vi "Oscilloscope Type Axis Scales.vi"(8 "Error In":errorcluster, 9 "Oscilloscope vertical":T1=[{"Volts/Div "=0.5, "Coupling"=enum."DC 1MOhm", "Offset [V]"=0.0, "Channel"=enum."Channel 1"}, {"Volts/Div "=0.2, "Coupling"=enum."DC 1MOhm", "Offset [V]"=0.0, "Channel"=enum."Channel 2"}] {"Offset [V]" format="%#_13p"; "Volts/Div" min=0.001 max=5.0 format="%#_6p"}, 11 "Graph In":refnum<vi>) -> (0 "Error Out":errorcluster, 3 "Graph Out":refnum<vi>)   [LabVIEW 2017]
uses:
  LC93xx HSN/LeC93xx Vertical.ctl
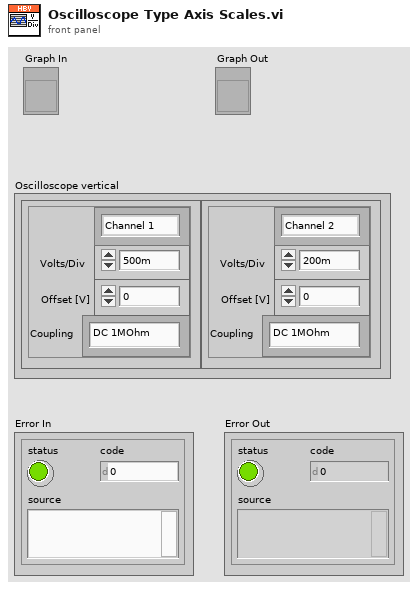
[diagram p1: front panel]
types:
  T1 = typedef "LeC93xx Vertical.ctl" = cluster{"Volts/Div ":dbl, "Coupling":enum16{"GND", "DC 50 Ohms", "DC 1MOhm", "AC 1MOhm"}, "Offset [V]":dbl, "Channel":enum16{"Channel 1", "Channel 2", "Channel 3", "Channel 4"}}[]
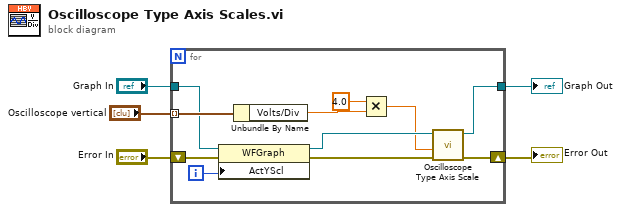
[diagram p0: block diagram]
diagram:
  n1 = for {
    shift-right: [w16] -> w5
    shift-left: "Error In" -> [w13]
    tunnel: "Oscilloscope vertical" -> [w15] mode=indexing
    tunnel: "Graph In" -> [w11]
    tunnel: [w14] -> w2
    i -> [w9]
    n2 = property class="WFGraph"(reference=w11, error in=w13, "ActYScl"=w9) -> (reference out=w10:refnum<vi>, error out=w12:errorcluster)
    n3 = Unbundle By Name(w15) -> ("Volts/Div"=w8:dbl)
    n4 = Multiply(x=4.0, y=w8) -> (x*y=w7:dbl)
    n5 = call "Oscilloscope Type Axis Scale.vi"("Error In"=w12, "Volts/Div"=w7, "Graph In"=w10) -> ("Error Out"=w16:errorcluster, "Graph Out"=w14:refnum<vi>)  [unwired: 7 in]
  }
  "Error Out" <- w5
  "Graph Out" <- w2
